vi "Set Initialization Data - ScopeSim.vi"(8 "error in":errorcluster, 11 "Head_ScopeSim in":refnum<class "Head_ScopeSim.lvclass">) -> (0 "error out":errorcluster, 3 "Head_ScopeSim out":refnum<class "Head_ScopeSim.lvclass">)   [LabVIEW 2019, in "Head_ScopeSim.lvclass"]
doc: "In this VI you can set the initialization data of a statically-linked subWorker."
uses:
  Head_ScopeSim.lvclass
  Scope Simulator/Initialization Data.ctl
  Scope Simulator/Response Cases.ctl
  <vilib>/addons/_Workers/Library/Case Label.ctl
  Head_ScopeSim.lvclass/Head_ScopeSim.ctl
  Scope Simulator/Scope Simulator.lvclass
  C:/Program Files (x86)/National Instruments/LabVIEW 2019/vi.lib/addons/_Workers/Library/Classes/Worker/Worker.lvclass
  <vilib>/addons/_Workers/Library/Workers.lvlib
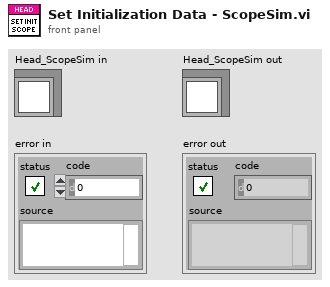
[diagram p1: front panel]
types:
  T1 = typedef "Scope Simulator.lvclass/Initialization Data.ctl" = cluster{"Response Cases":T2}
  T2 = typedef "Scope Simulator.lvclass/Response Cases.ctl" = cluster{"Generated Waveform":T3, "Scope Status":T3}
  T3 = typedef "Workers.lvlib/Case Label.ctl" = string
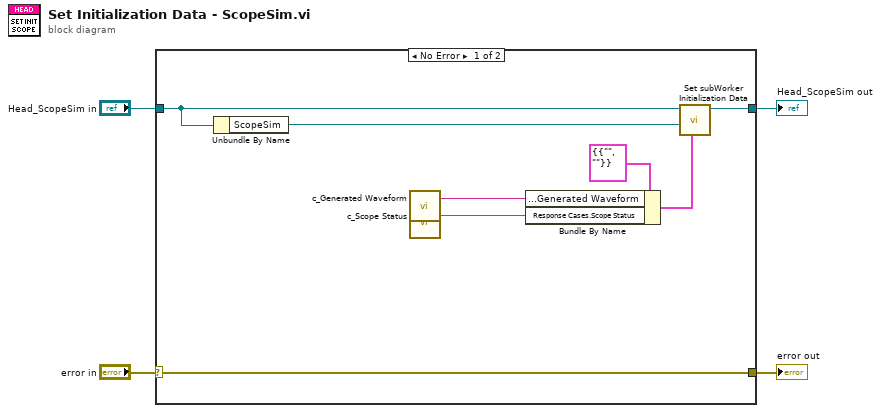
[diagram p0: block diagram]
diagram:
  n1 = case shown="No Error" "error in" {
    selector: "error in" -> [w12 w14]
    tunnel: [w12 w14] -> w3
    tunnel: [w10 w13] -> w2
    tunnel: "Head_ScopeSim in" -> [w9 w13]
    frame No Error {
      n2 = Unbundle By Name(w9) -> ("ScopeSim"=w11:refnum<class "Scope Simulator.lvclass">)
      n3 = call "c_Generated Waveform.vi"() -> ("Case Label"=w5:T3)  [unwired: 1 in]
      n4 = call "c_Scope Status.vi"() -> ("Case Label"=w6:T3)  [unwired: 1 in]
      n5 = Bundle By Name(cluster=T1 {"Response Cases"={"Generated Waveform"="", "Scope Status"=""}} ("Initialization Data"), "Response Cases.Generated Waveform"=w5, "Response Cases.Scope Status"=w6) -> (w7:T1)
      n6 = call-dynamic "Set subWorker Initialization Data.vi"("Initialization Data"=w7, "subWorker"=w11, "Worker"=w9) -> ("Worker out"=w10:refnum<class "Head_ScopeSim.lvclass">)  [unwired: 8 in]
    }
    frame Error {
    }
  }
  "error out" <- w3
  "Head_ScopeSim out" <- w2
